vi "Set Project Path.vi"(10 "Project Path":path, 11 "CD Build Tools in":refnum<class "Project Build Tools.lvclass">) -> (3 "CD Build Tools out":refnum<class "Project Build Tools.lvclass">)   [LabVIEW 2019, in "Project Build Tools.lvclass"]
uses:
  Project Build Tools.lvclass
  Project Build Tools.lvclass/Project Build Tools.ctl
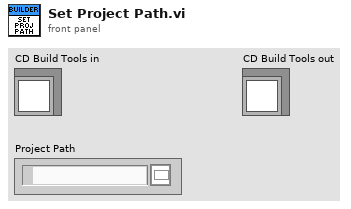
[diagram p1: front panel]
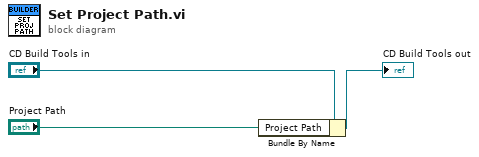
[diagram p0: block diagram]
diagram:
  n1 = Bundle By Name(cluster="CD Build Tools in", "Project Path"="Project Path") -> (→"CD Build Tools out":refnum<class "Project Build Tools.lvclass">)
